vi "robot - Lighted Circle.vi"(6 "Lowered":bool, 8 "Light Direction":dbl(knob)=314.8880943229338 scale=0.0..360.0 scale format="%.1f", 9 "Color":u32(colorbox)=13395558, 10 "Pict Rect":T1={"left"=20, "top"=20, "right"=50, "bottom"=50}, 11 "Picture In":picture) -> (3 "Picture Out":picture)   [LabVIEW 2023]
doc: "This VI draws an oval in two shades of color to give the look of depth. (Light direction is specified in degrees.)"
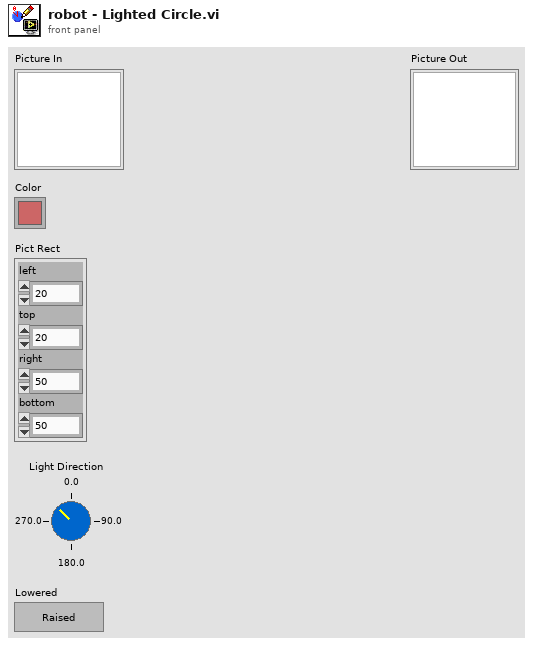
[diagram p1: front panel]
types:
  T1 = cluster{"left":i16, "top":i16, "right":i16, "bottom":i16}
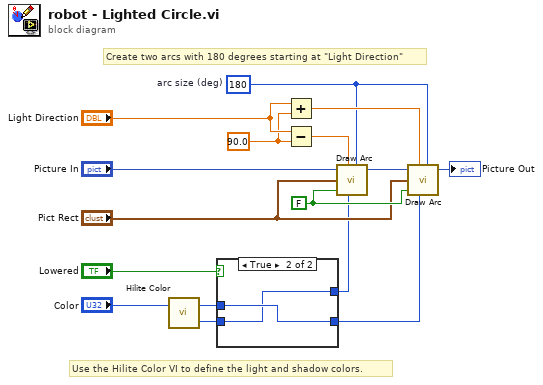
[diagram p0: block diagram]
diagram:
  w1 = 90.0
  w2 = 180  # arc size (deg)
  w15 = FALSE
  # "Use the Hilite Color VI to define the light and shadow colors."
  # "Create two arcs with 180 degrees starting at \"Light Direction\""
  n1 = call <vilib>:"Hilite Color.vi"("Color In"="Color") -> ("Shadow"=w6:u32, "Hilite"=w7:u32)  [unwired: 1 in]
  n2 = case shown="True" "Lowered" {
    tunnel: w7 -> [w17 w20]
    tunnel: w6 -> [w18 w19]
    tunnel: [w18 w20] -> w5
    tunnel: [w17 w19] -> w4
    frame False {
    }
    frame True {
    }
  }
  n3 = Add(x="Light Direction", y=w1) -> (x+y=w9:dbl)
  n4 = Subtract(x="Light Direction", y=w1) -> (x-y=w11:dbl)
  n5 = call <vilib>:"Draw Arc.vi"("picture"="Picture In", "start angle[degrees]"=w11, "rect"="Pict Rect", "fill?(F)"=w15, "color(black)"=w4, "arc size[degrees]"=w2) -> ("new picture"=w16:picture)  [unwired: 3 in]
  n6 = call <vilib>:"Draw Arc.vi"("picture"=w16, "start angle[degrees]"=w9, "rect"="Pict Rect", "fill?(F)"=w15, "color(black)"=w5, "arc size[degrees]"=w2) -> ("new picture"=→"Picture Out":picture)  [unwired: 3 in]
